vi "UE9 Stream Example LJ_swSLEEP.vi"() -> ()   [LabVIEW 2021]
panel:
  in  "Simulated Processing Delay [ms]":u32
  out "UD Backlog [%]":dbl format="%.2f"
  in  "AIN Range":u16(ring) items=["LJ_rgBIP5V", "LJ_rgUNI5V", "LJ_rgUNI2P5V", "LJ_rgUNI1P25V", "LJ_rgUNIP625V"]
  in  "Scan List":u8[](array[numeric])=[0, 1, 2, 3]
  out "Actual Scan Rate (Hz)":dbl=1000.0 format="%.3f"
  out "ms Per Loop":u32
  out "Comm Backlog [%]":dbl format="%.2f"
  out "Scans Retrieved Sec (measured)":dbl format="%.2f"
  out "# Scans Read":i32
  out "# of iterations":i32
  out "Data":dbl[][](array[numeric]) format="%.3f"
  in  "Scan Rate (Hz)":dbl=1000.0 format="%.3f"
  in  "Data File Extension":string="dat"
  out "Current Data File":path
  in  "Data File Prefix":string="data"
  in  "Write To File":bool
  in  "FirstFound":bool=TRUE
  in  "stop":bool
  in  "ConnectionType":u16(ring) items=["LJ_ctUSB", "LJ_ctETHERNET"]
  in  "DeviceType":u16(ring)=1 items=["LJ_dtU3", "LJ_dtUE9"]
  in  "Address":string="192.168.1.209"
  out "Error Message":string
  in  "Resolution":i32=12
  # "The actual scans/sec is controlled\nby hardware and is known.  This\n\"measured\" suggests the rate at\nwhich data is being retreived."
  # "Specify an IP address for Ethernet, or Local ID\nfor USB.  If FirstFound is selected, Local ID is\nignored for USB.  Clear FirstFound if using Ethernet."
  # "(for all channels)"
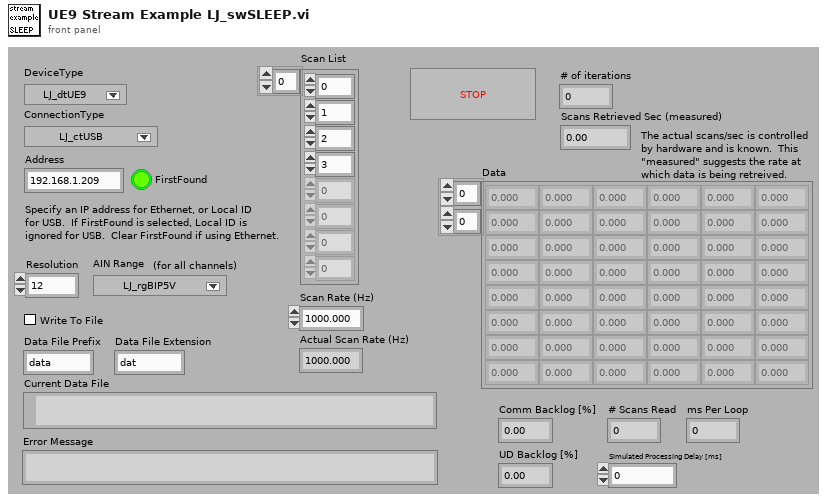
[diagram p1: front panel]
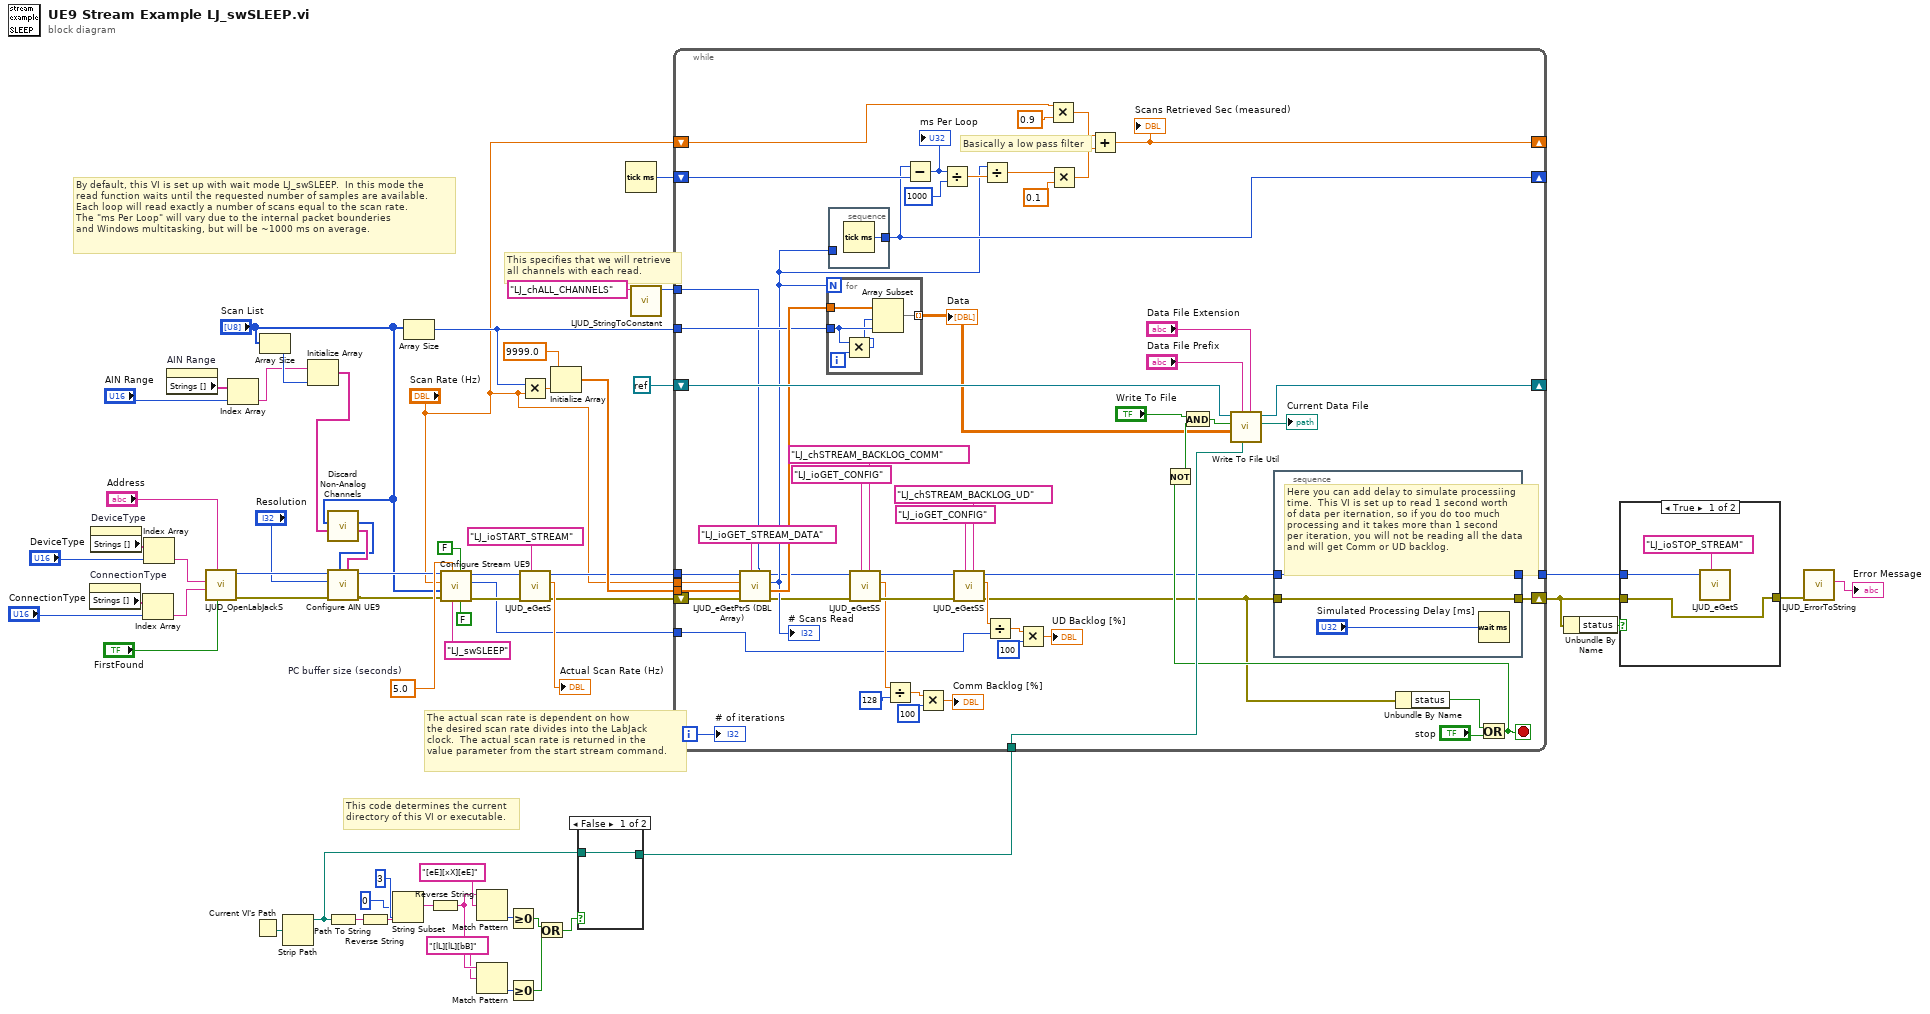
[diagram p0: block diagram]
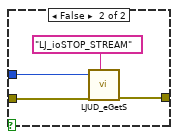
[diagram p2: hidden frame]
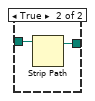
[diagram p3: hidden frame]
diagram:
  w31 = 5.0  # PC buffer size (seconds)
  # "This specifies that we will retrieve\nall channels with each read."
  # "The actual scan rate is dependent on how\nthe desired scan rate divides into the LabJack\nclock.  The actual scan rate is returned in the\nvalue parameter from the start stream command."
  # "By default, this VI is set up with wait mode LJ_swSLEEP.  In this mode the\nread function waits until the requested number of samples are available.\nEach loop will read exactly a number of scans equal to the scan rate.\nThe \"ms Per Loop\" will vary due to the internal packet bounderies\nand Windows multitasking, but will be ~1000 ms on average."
  # "This code determines the current\ndirectory of this VI or executable."
  n1 = property on="ConnectionType" class="Ring (strict)"() -> ("Strings []"=w15:string[])  [unwired: 2 in, 2 out]
  n2 = property on="DeviceType" class="Ring (strict)"() -> ("Strings []"=w16:string[])  [unwired: 2 in, 2 out]
  n3 = Index Array(array=w15, index="ConnectionType") -> (element=w11:string)
  n4 = Index Array(array=w16, index="DeviceType") -> (element=w12:string)
  n5 = property on="AIN Range" class="Ring (strict)"() -> ("Strings []"=w18:string[])  [unwired: 2 in, 2 out]
  n6 = call "LJUD_OpenLabJackS.vi"("FirstFound"="FirstFound", "Address"="Address", "ConnectionType"=w11, "DeviceType"=w12) -> ("error out"=w25:errorcluster, "Handle"=w24:i32)  [unwired: 5 in, 1 out]
  n7 = Index Array(array=w18, index="AIN Range") -> (element=w19:string)
  n8 = Current VI's Path() -> (path=w59:path)
  n9 = Array Size(array="Scan List") -> (size(s)=w22:i32)
  n10 = Strip Path(path=w59) -> (stripped path=w51:path)  [unwired: 1 out]
  n11 = Initialize Array(w19, w22) -> (w7:string[])
  n12 = call "Discard Non-Analog Channels.vi"("Ranges In"=w7, "Channels In"="Scan List") -> ("Ranges Out"=w5:string[], "Channels Out"=w4:i32[])  [unwired: 6 in, 2 out]
  n13 = call "Configure AIN UE9.vi"("Ranges"=w5, "Channels"=w4, "error in"=w25, "Resolution"="Resolution", "Handle In"=w24) -> ("error out"=w27:errorcluster, "Handle Out"=w26:i32)  [unwired: 5 in]
  n14 = Path To String(path=w51) -> (string=w58:string)
  n15 = Reverse String(1:w58) -> (0:w57:string)
  n16 = String Subset(string=w57, offset (0)=0, length (rest)=3 ("length")) -> (substring=w54:string)
  n17 = Array Size(array="Scan List") -> (size(s)=w37:i32)
  n18 = Reverse String(1:w54) -> (0:w50:string)
  n19 = call "Configure Stream UE9.vi"("External Scan Trigger"=FALSE, "Scan Clock Output"=FALSE, "Wait Mode"="LJ_swSLEEP" ("Wait Mode (2)"), "PC buffer size (seconds)"=w31, "error in"=w27, "Scan List"="Scan List", "Scan Rate (Hz)"="Scan Rate (Hz)", "Handle In"=w26) -> ("error out"=w41:errorcluster, "PC buffer size (samples)"=w1:i32, "Handle Out"=w42:i32)  [unwired: 1 in]
  n20 = Match Pattern(string=w50, regular expression="[eE][xX][eE]") -> (offset past match=w52:i32)  [unwired: 1 in, 3 out]
  n21 = Match Pattern(string=w50, regular expression="[lL][lL][bB]") -> (offset past match=w47:i32)  [unwired: 1 in, 3 out]
  n22 = Greater Or Equal To 0?(x=w52) -> (x >= 0?=w48:bool)
  n23 = Greater Or Equal To 0?(x=w47) -> (x >= 0?=w46:bool)
  n24 = Multiply(x=w37, y="Scan Rate (Hz)") -> (x*y=w40:dbl)
  n25 = call "LJUD_eGetS.vi"("IOType"="LJ_ioSTART_STREAM", "error in"=w41, "Handle In"=w42) -> ("error out"=w3:errorcluster, "Value Read"=→"Actual Scan Rate (Hz)":dbl, "Handle Out"=w21:i32)  [unwired: 6 in]
  n26 = Or(x=w48, y=w46) -> (x .or. y?=w45:bool)
  n27 = Initialize Array(9999.0, w40) -> (w38:dbl[])
  n28 = case shown="False" w45 {
    tunnel: w51 -> [w63 w65]
    tunnel: [w63 w64] -> w44
    frame False {
    }
    frame True {
      n29 = Strip Path(path=w65) -> (stripped path=w64:path)  [unwired: 1 out]
    }
  }
  n30 = Tick Count (ms)() -> (millisecond timer value=w32:u32)
  n31 = call "LJUD_StringToConstant.vi"("String"="LJ_chALL_CHANNELS") -> ("Constant Number"=w8:i32)  [unwired: 9 in, 1 out]
  n32 = while {
    tunnel: w1 -> [w72]
    shift-left: w3 -> [w80]
    shift-right: [w68] -> w2
    tunnel: w8 -> [w85]
    shift-left: "Scan Rate (Hz)" -> [w94]
    shift-right: [w91] -> _
    shift-left: w32 -> [w103]
    shift-right: [w100] -> _
    tunnel: [w66] -> w35
    tunnel: w37 -> [w105]
    tunnel: w38 -> [w108]
    tunnel: "Scan Rate (Hz)" -> [w106]
    tunnel: w44 -> [w112]
    shift-left: refnum<k0> refnum -> [w118]
    shift-right: [w117] -> _
    tunnel: w21 -> [w110]
    i -> [w104]
    stop <- w111 stop-if-true
    # "Basically a low pass filter"
    n33 = call "LJUD_eGetPtrS (DBL Array).vi"("Channel"=w85, "IOType"="LJ_ioGET_STREAM_DATA", "error in"=w80, "DBL Array Write"=w108, "Value"=w106, "Handle In"=w110) -> ("error out"=w89:errorcluster, "DBL Array Read"=w107:dbl[], "Value"=w98:i32, "Handle Out"=w90:i32)  [unwired: 2 in]
    "# Scans Read" <- w98
    n34 = for {
      N: w98 -> [_]
      tunnel: w107 -> [w131]
      tunnel: w105 -> [w130]
      tunnel: [w127] -> w86 mode=indexing
      i -> [w129]
      n35 = Multiply(x=w130, y=w129) -> (x*y=w128:i32)
      n36 = Array Subset(array=w131, index=w128, length=w130) -> (w127:dbl[])
    }
    "Data" <- w86
    n37 = stacked-sequence {
      tunnel: w98 -> [_]
      tunnel: [w126] -> w100
      frame #0 {
        n38 = Tick Count (ms)() -> (millisecond timer value=w126:u32)
      }
    }
    n39 = call "LJUD_eGetSS.vi"("Channel"="LJ_chSTREAM_BACKLOG_COMM", "IOType"="LJ_ioGET_CONFIG", "error in"=w89, "Handle In"=w90) -> ("error out"=w81:errorcluster, "Value Read"=w76:dbl, "Handle Out"=w82:i32)  [unwired: 5 in]
    n40 = Divide(x=w76, y=128) -> (x/y=w79:dbl)
    n41 = Subtract(x=w100, y=w103) -> (x-y=w102:u32)
    "ms Per Loop" <- w102
    n42 = Multiply(x=w79, y=100) -> (x*y=→"Comm Backlog [%]":dbl)
    n43 = Divide(x=w102, y=u32 1000) -> (x/y=w99:dbl)
    n44 = call "LJUD_eGetSS.vi"("Channel"="LJ_chSTREAM_BACKLOG_UD", "IOType"="LJ_ioGET_CONFIG", "error in"=w81, "Handle In"=w82) -> ("error out"=w69:errorcluster, "Value Read"=w71:dbl, "Handle Out"=w67:i32)  [unwired: 5 in]
    n45 = Divide(x=w98, y=w99) -> (x/y=w97:dbl)
    n46 = Divide(x=w71, y=w72) -> (x/y=w73:dbl)
    n47 = Multiply(x=w73, y=100) -> (x*y=→"UD Backlog [%]":dbl)
    n48 = Multiply(x=w94, y=0.9) -> (x*y=w93:dbl)
    n49 = Multiply(x=w97, y=0.1) -> (x*y=w92:dbl)
    n50 = Add(x=w93, y=w92) -> (x+y=w91:dbl)
    "Scans Retrieved Sec (measured)" <- w91
    n51 = stacked-sequence {
      tunnel: w69 -> [w125]
      tunnel: [w125] -> w68
      tunnel: w67 -> [w124]
      tunnel: [w124] -> w66
      frame #0 {
        # "Here you can add delay to simulate processiing\ntime.  This VI is set up to read 1 second worth\nof data per iternation, so if you do too much\nprocessing and it takes more than 1 second\nper iteration, you will not be reading all the data\nand will get Comm or UD backlog."
        n52 = Wait (ms)(milliseconds to wait="Simulated Processing Delay [ms]") -> ()  [unwired: 1 out]
      }
    }
    n53 = Unbundle By Name(w69) -> ("status"=w121:bool)
    n54 = Or(x=w121, y="stop") -> (x .or. y?=w111:bool)
    n55 = Not(x=w111) -> (.not. x?=w113:bool)
    n56 = And(x="Write To File", y=w113) -> (x .and. y?=w114:bool)
    n57 = call "Write To File Util.vi"("Data File Extension"="Data File Extension", "Working Directory"=w112, "Data File Prefix"="Data File Prefix", "Data"=w86, "Write To File"=w114, "File Refnum In"=w118) -> ("Current Data File"=→"Current Data File":path, "File Refnum Out"=w117:refnum<file>)  [unwired: 3 in, 1 out]
    "# of iterations" <- w104
  }
  n58 = Unbundle By Name(w2) -> ("status"=w10:bool)
  n59 = case shown="True" w10 {
    tunnel: w35 -> [w133 w137]
    tunnel: [w132 w136] -> w34
    tunnel: w2 -> [w132 w135]
    frame True {
      n60 = call "LJUD_eGetS.vi"("IOType"="LJ_ioSTOP_STREAM", "Handle In"=w133) -> ()  [unwired: 7 in, 3 out]
    }
    frame False {
      n61 = call "LJUD_eGetS.vi"("IOType"="LJ_ioSTOP_STREAM", "error in"=w135, "Handle In"=w137) -> ("error out"=w136:errorcluster)  [unwired: 6 in, 2 out]
    }
  }
  n62 = call "LJUD_ErrorToString.vi"("error in"=w34) -> ("String"=→"Error Message":string)  [unwired: 10 in]
